vi "calc.vi"(11 "Qube":refnum<class "System.lvclass">) -> (3 "Qube":refnum<class "System.lvclass">)   [LabVIEW 2021, in "System.lvclass"]
uses:
  System.lvclass
  System.lvclass/System.ctl
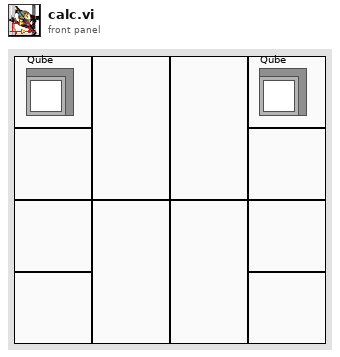
[diagram p1: front panel]
types:
  T1 = typedef "System.lvclass/mode.ctl" = enum16{"pry_OL", "pry_CL", "FBLR_CL"}
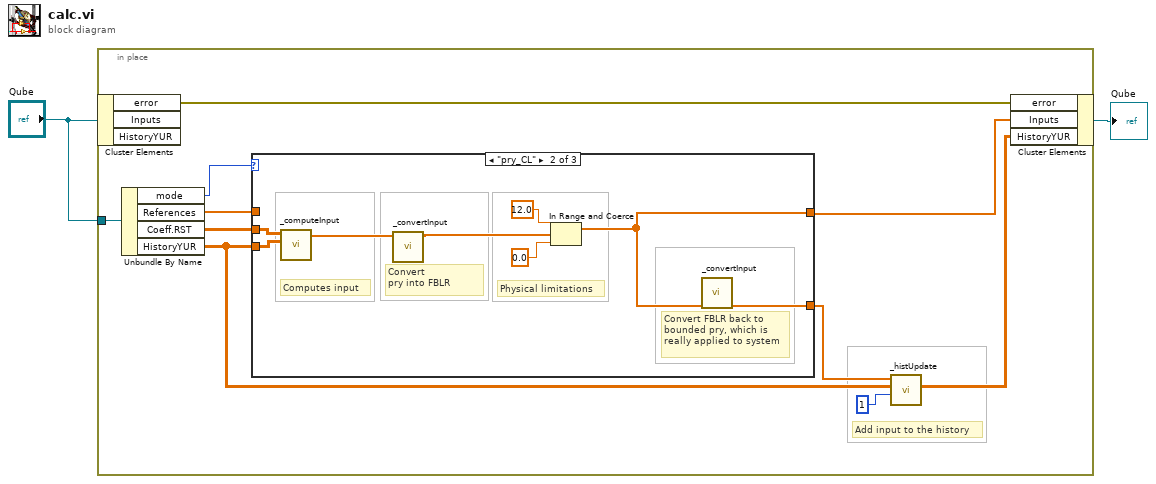
[diagram p0: block diagram]
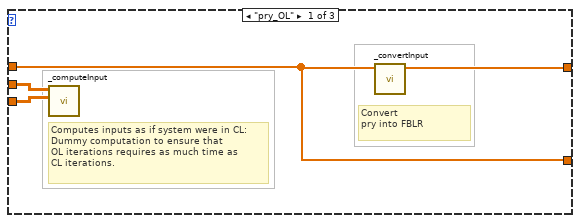
[diagram p2: hidden frame]
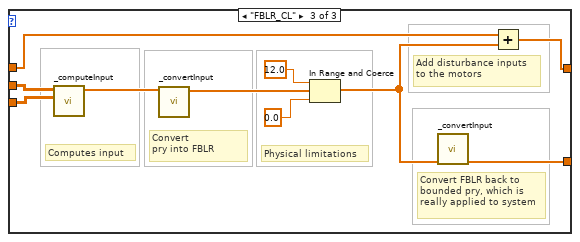
[diagram p3: hidden frame]
diagram:
  n1 = in-place {
    in-place-border: "Qube" -> [w11]
    # "Add input to the history"
    n2 = in-place-cluster #1("Qube") -> ("error"=w12:errorcluster)  [unwired: 2 out]
    n3 = Unbundle By Name(w11) -> ("mode"=w10:T1, "References"=w9:dbl[], "Coeff.RST"=w8:dbl[][][], "HistoryYUR"=w6:dbl[][][])
    n4 = case shown="\"pry_CL\"" w10 {
      tunnel: [w13 w17 w28] -> w5
      tunnel: w9 -> [w13 _ w29]
      tunnel: w8 -> [w16 w24 w34]
      tunnel: w6 -> [w15 w23 w33]
      tunnel: [w14 w18 w30] -> w4
      frame "pry_OL" {
        # "Convert \npry into FBLR"
        # "Computes inputs as if system were in CL:\nDummy computation to ensure that\nOL iterations requires as much time as\nCL iterations."
        n5 = call "_computeInput.vi"("HistoryYUR"=w15, "Coeff.RST"=w16) -> ()  [unwired: 9 in, 1 out]
        n6 = call "_convertInput.vi"("pry"=w13) -> ("FBLR"=w14:dbl[])  [unwired: 8 in, 1 out]
      }
      frame "pry_CL" {
        # "Convert FBLR back to\nbounded pry, which is \nreally applied to system"
        # "Physical limitations"
        # "Convert \npry into FBLR"
        # "Computes input"
        n7 = call "_computeInput.vi"("HistoryYUR"=w23, "Coeff.RST"=w24) -> ("u"=w20:dbl[])  [unwired: 9 in]
        n8 = call "_convertInput.vi"("pry"=w20) -> ("FBLR"=w19:dbl[])  [unwired: 8 in, 1 out]
        n9 = In Range and Coerce(upper limit=12.0 ("y"), x=w19, lower limit=0.0 ("y")) -> (coerced(x)=w18:dbl[])  [unwired: 1 out]
        n10 = call "_convertInput.vi"("FBLR"=w18) -> ("pry"=w17:dbl[])  [unwired: 8 in, 1 out]
      }
      frame "FBLR_CL" {
        # "Computes input"
        # "Convert \npry into FBLR"
        # "Physical limitations"
        # "Add disturbance inputs\nto the motors"
        # "Convert FBLR back to\nbounded pry, which is \nreally applied to system"
        n11 = call "_computeInput.vi"("HistoryYUR"=w33, "Coeff.RST"=w34) -> ("u"=w26:dbl[])  [unwired: 9 in]
        n12 = call "_convertInput.vi"("pry"=w26) -> ("FBLR"=w25:dbl[])  [unwired: 8 in, 1 out]
        n13 = In Range and Coerce(upper limit=12.0 ("y"), x=w25, lower limit=0.0 ("y")) -> (coerced(x)=w27:dbl[])  [unwired: 1 out]
        n14 = call "_convertInput.vi"("FBLR"=w27) -> ("pry"=w28:dbl[])  [unwired: 8 in, 1 out]
        n15 = Add(x=w29, y=w27) -> (x+y=w30:dbl[])
      }
    }
    n16 = call "_histUpdate.vi"("Y:0-U:1-R:2"=1, "History In"=w6, "pry"=w5) -> ("History Out"=w3:dbl[][][])  [unwired: 8 in]
    n17 = in-place-cluster #1("error"=w12, "Inputs"=w4, "HistoryYUR"=w3) -> (→"Qube":refnum<class "System.lvclass">)
  }
